vi "extract_para_from_command.vi"(8 "error in (no error)":errorcluster, 11 "Instrument Command In":string=":ACP:OFFS{1|2}:LIST:RCAR {<REAL>}, {<REAL>}, {<REAL>}, {<REAL>}, {<REAL>}, {<REAL>}") -> (0 "error out":errorcluster, 2 "Auto Extracted Contol Specs":T1, 3 "Instrument Command In Out":string)   [LabVIEW 2018]
uses:
  TypeDefinitions/auto_extracted_control_specs.ctl
  TypeDefinitions/auto_extracted_control_spec.ctl
  Gtor/Mth/GenVI/Intf/GenStdVI/Mth/GenOneStdVI/TypeDefinitions/control_data_type.ctl
  Gtor/Mth/GenVI/Intf/GenStdVI/Mth/GenOneStdVI/TypeDefinitions/control_class.ctl
  Gtor/Mth/GenVI/Intf/GenStdVI/Mth/GenOneStdVI/TypeDefinitions/ring_string_and_value.ctl
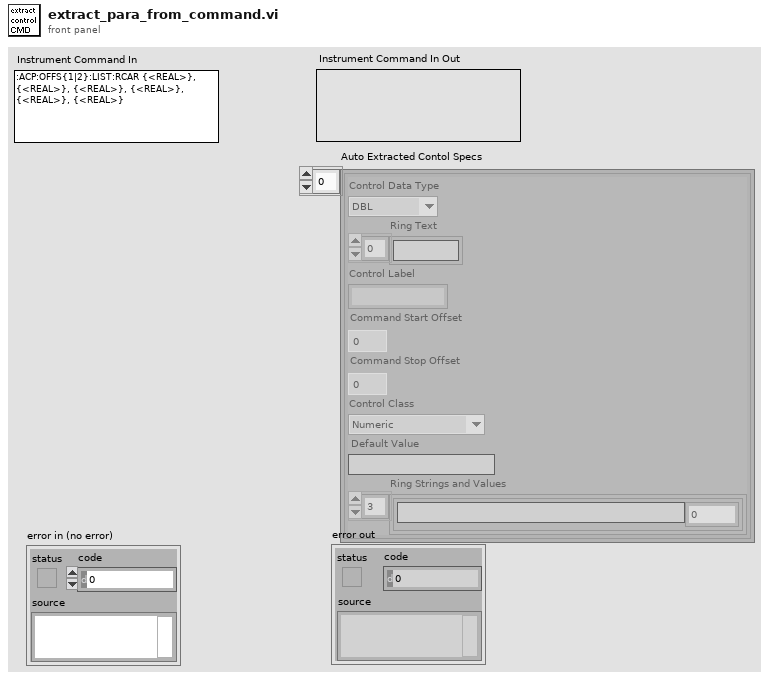
[diagram p1: front panel]
types:
  T1 = typedef "auto_extracted_control_specs.ctl" = T2[]
  T2 = typedef "auto_extracted_control_spec.ctl" = cluster{"Control Data Type":T3, "Ring Text":string[], "Control Label":string, "Command Start Offset":i32, "Command Stop Offset":i32, "Control Class":T4, "Default Value":string, "Ring Strings and Values":T5[]}
  T3 = typedef "control_data_type.ctl" = enum16{"DBL", "I32", "Boolean", "String", "U16", "U32", "EXT", "SGL", "I16", "U8", "I8", "I64", "U64", "Waveform", "Reference", "Variant", "Cluster"}
  T4 = typedef "control_class.ctl" = enum16{"Numeric", "Vertical Slide Switch", "Text Ring", "String", "Array", "VISAName", "WaveformGraph", "Cluster"}
  T5 = typedef "ring_string_and_value.ctl" = cluster{"String":string, "Value":dbl}
  T6 = cluster{"Start Sting":string, "End String":string}
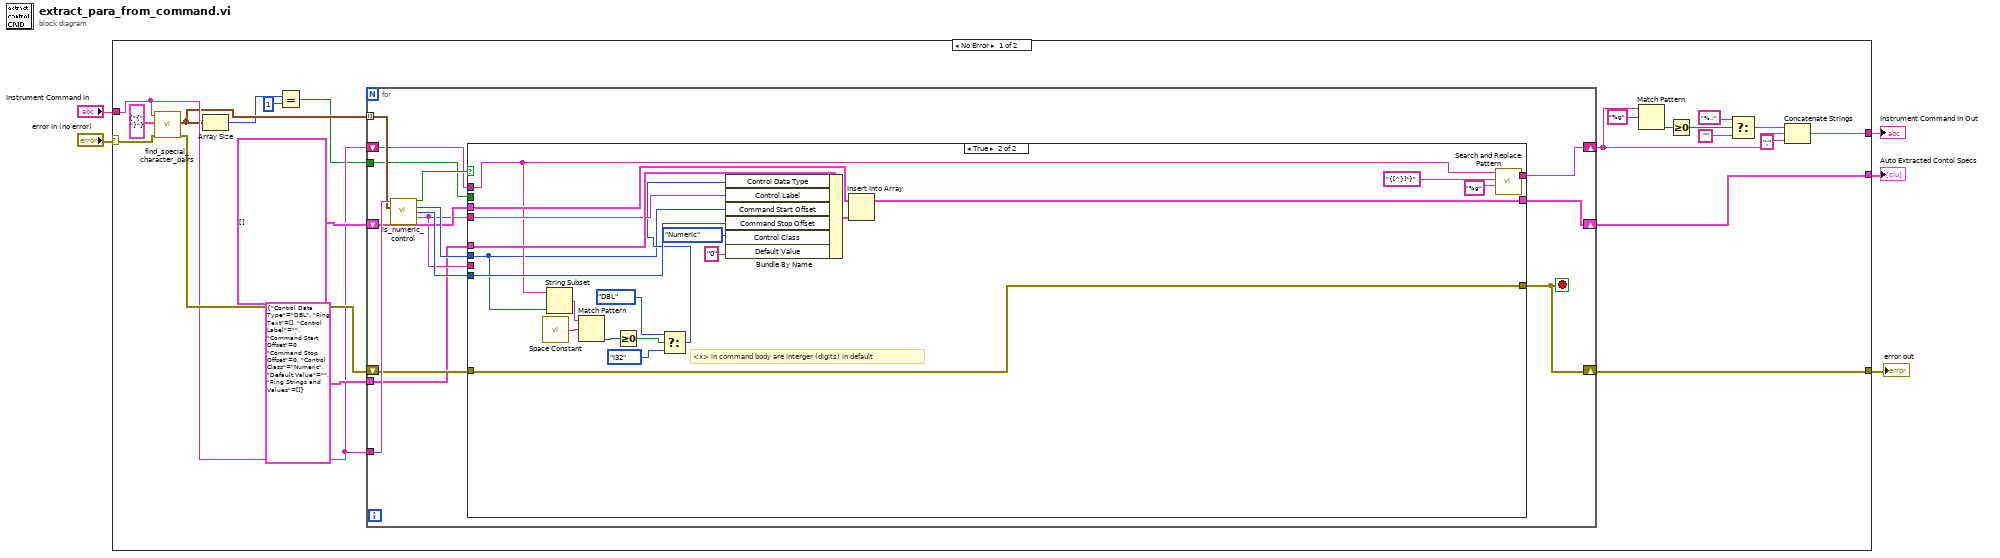
[diagram p0: block diagram]
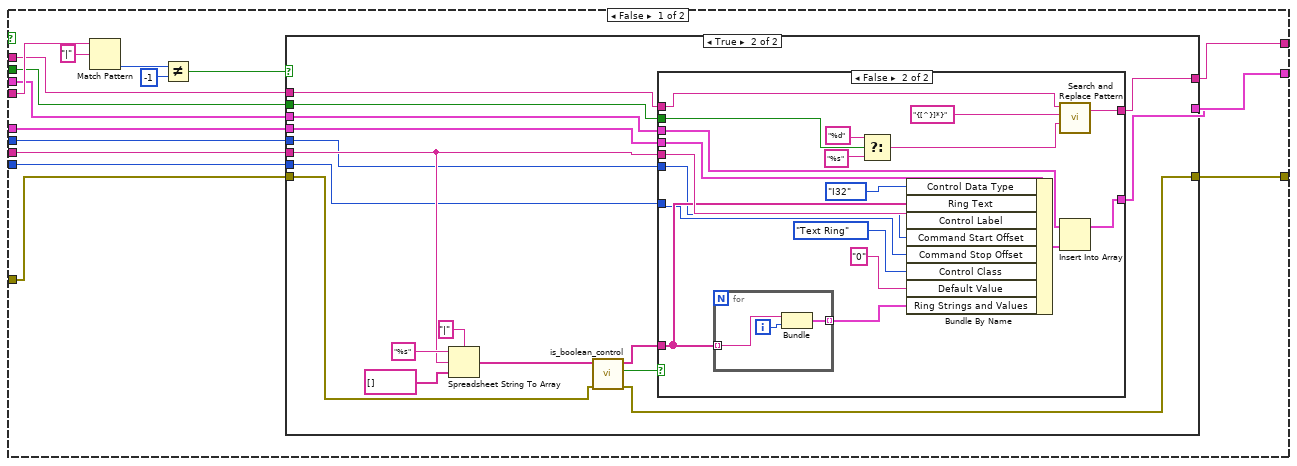
[diagram p2: hidden frame]
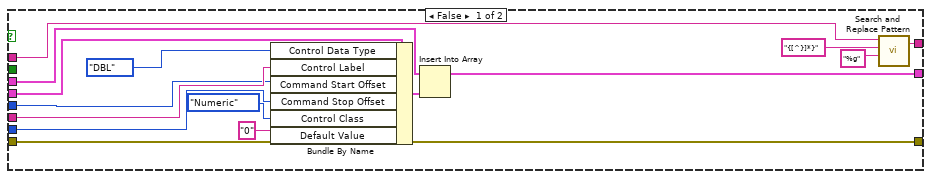
[diagram p3: hidden frame]
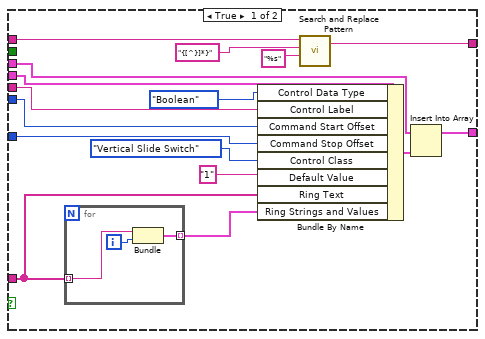
[diagram p4: hidden frame]
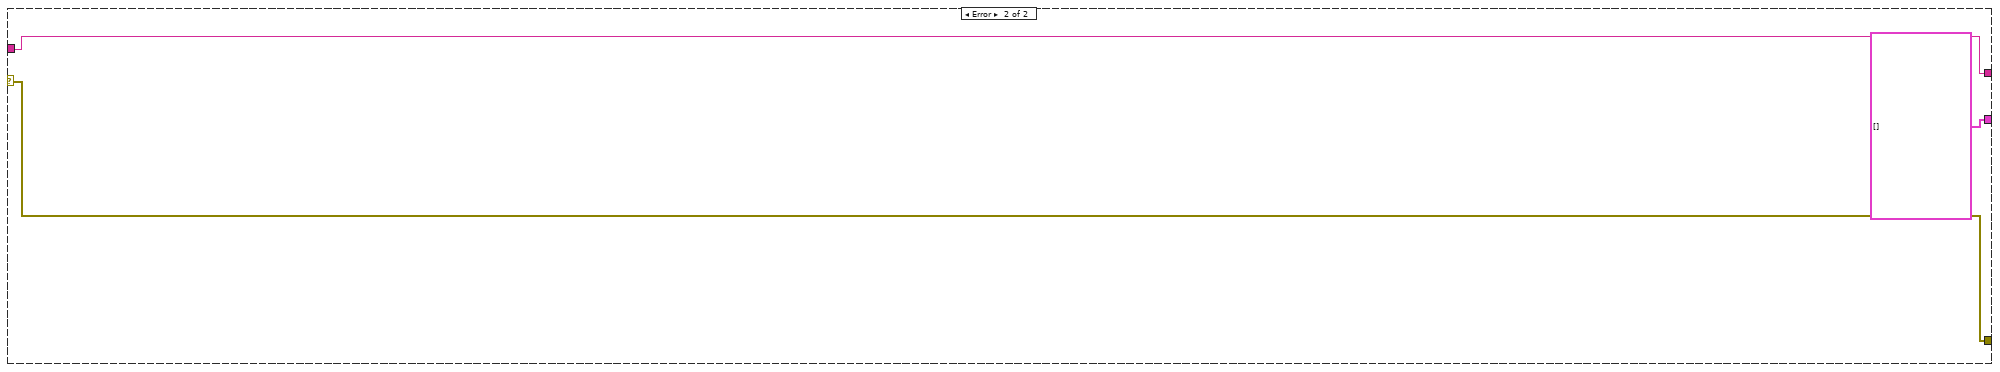
[diagram p5: hidden frame]
diagram:
  n1 = case shown="No Error" "error in (no error)" {
    selector: "error in (no error)" -> [w22 w153]
    tunnel: "Instrument Command In" -> [w19 w151]
    tunnel: [w24 T1 [] ("Auto Extracted Contol Specs")] -> w5
    tunnel: [w23 w153] -> w2
    tunnel: [w11 w151] -> w1
    frame No Error {
      n2 = call "find_special_character_pairs.vi"("error in (no error)"=w22, "String Pair"=T6 {"Start Sting"="{", "End String"="}"}, "Command String"=w19) -> ("error out"=w21:errorcluster, "Pair Offset"=w10:cluster{"Start Offset":i32, "End offset":i32}[])  [unwired: 7 out]
      n3 = Array Size(array=w10) -> (size(s)=w9:i32)
      n4 = Equal?(x=w9, y=1) -> (x = y?=w7:bool)
      n5 = for {
        tunnel: w10 -> [w39] mode=indexing
        tunnel: w19 -> [w40]
        shift-right: [w34] -> w24
        shift-left: T1 [] ("Auto Extracted Contol Specs") -> [w35]
        shift-right: [w27] -> w23
        shift-left: w21 -> [w32]
        tunnel: T2 {"Control Data Type"=enum."DBL", "Ring Text"=[], "Control Label"="", "Command Start Offset"=0, "Command Stop Offset"=0, "Control Class"=enum."Numeric", "Default Value"="", "Ring Strings and Values"=[]} ("Auto Extracted Contol Spec") -> [w31]
        shift-right: [w29] -> w12
        shift-left: w19 -> [w30]
        tunnel: w7 -> [w28]
        stop <- w27 stop-if-true
        n6 = call "is_numeric_control.vi"("Polished Command In"=w40, "Cluster"=w39) -> ("Is Numeric"=w38:bool, "Start Offset"=w37:i32, "End offset"=w36:i32, "Parameter Strings"=w33:string)  [unwired: 1 in, 9 out]
        n7 = case shown="True" w38 {
          tunnel: w33 -> [w55 w146]
          tunnel: w37 -> [w50 w130]
          tunnel: w36 -> [w49 w142]
          tunnel: w35 -> [w48 w150]
          tunnel: [w47 w149] -> w34
          tunnel: w33 -> [w51 _]
          tunnel: w32 -> [w46 w148]
          tunnel: [w45 w148] -> w27
          tunnel: w31 -> [w41 w147]
          tunnel: w30 -> [w44 w133]
          tunnel: [w43 w139] -> w29
          tunnel: w28 -> [w42 _]
          frame False {
            n8 = Match Pattern(string=w55, regular expression="|") -> (offset past match=w54:i32)  [unwired: 4 out]
            n9 = Not Equal?(x=w54, y=-1) -> (x != y?=w52:bool)
            n10 = case shown="True" w52 {
              tunnel: w51 -> [w68 w83]
              tunnel: w50 -> [w59 w82]
              tunnel: w49 -> [w63 w81]
              tunnel: w48 -> [w71 w84]
              tunnel: [w70 w80] -> w47
              tunnel: w46 -> [w69 w78]
              tunnel: [w69 w77] -> w45
              tunnel: w41 -> [w65 w76]
              tunnel: w44 -> [w58 w75]
              tunnel: [w60 w74] -> w43
              tunnel: w42 -> [_ w73]
              frame False {
                n11 = Bundle By Name(cluster=w65, "Control Data Type"=control_data_type."DBL", "Control Label"=w68, "Command Start Offset"=w59, "Command Stop Offset"=w63, "Control Class"=control_class."Numeric", "Default Value"="0") -> (w64:T2)
                n12 = Insert Into Array(array=w71, new element=w64) -> (w70:T1)  [unwired: 1 in]
                n13 = call <vilib>:"Search and Replace Pattern.vi"("string"=w58, "regular expression (\"\")"="{[^}]*}" ("substring (\"\")"), "replace string (\"\")"="%g" ("substring (\"\")")) -> ("result string"=w60:string)  [unwired: 3 out]
              }
              frame True {
                n14 = Spreadsheet String To Array(delimiter (Tab)="|", format string="%s" ("spreadsheet string"), spreadsheet string=w83, array type (2D Dbl)=string[] []) -> (array=w79:string[])
                n15 = call "is_boolean_control.vi"("error in (no error)"=w78, "CMD Ring Value"=w79) -> ("error out"=w77:errorcluster, "Is Boolean"=w85:bool, "CMD Ring Value Out"=w72:string[])  [unwired: 7 out]
                n16 = case shown="False" w85 {
                  tunnel: w84 -> [w104 w126]
                  tunnel: w83 -> [w100 w122]
                  tunnel: w82 -> [w95 w115]
                  tunnel: w81 -> [w96 w116]
                  tunnel: [w103 w125] -> w80
                  tunnel: w72 -> [w90 w120]
                  tunnel: w76 -> [w102 w124]
                  tunnel: w75 -> [w93 w114]
                  tunnel: [w91 w112] -> w74
                  tunnel: w73 -> [_ w111]
                  frame True {
                    n17 = for {
                      tunnel: w90 -> [w107] mode=indexing
                      tunnel: [w105] -> w89 mode=indexing
                      i -> [w106]
                      n18 = Bundle("Ring Value"=w107, w106) -> (w105:cluster{"Ring Value":string, i32})  [unwired: 1 out]
                    }
                    n19 = Bundle By Name(cluster=w102, "Control Data Type"=control_data_type."Boolean", "Control Label"=w100, "Command Start Offset"=w95, "Command Stop Offset"=w96, "Control Class"=control_class."Vertical Slide Switch", "Default Value"="1", "Ring Text"=w90, "Ring Strings and Values"=w89) -> (w98:T2)
                    n20 = call <vilib>:"Search and Replace Pattern.vi"("string"=w93, "regular expression (\"\")"="{[^}]*}" ("substring (\"\")"), "replace string (\"\")"="%s" ("substring (\"\")")) -> ("result string"=w91:string)  [unwired: 3 out]
                    n21 = Insert Into Array(array=w104, new element=w98) -> (w103:T1)  [unwired: 1 in]
                  }
                  frame False {
                    n22 = for {
                      tunnel: w120 -> [w129] mode=indexing
                      tunnel: [w127] -> w119 mode=indexing
                      i -> [w128]
                      n23 = Bundle("Ring Value"=w129, w128) -> (w127:cluster{"Ring Value":string, i32})  [unwired: 1 out]
                    }
                    n24 = Select(t="%d" ("substring (\"\")"), s=w111, f="%s") -> (s? t:f=w109:string)
                    n25 = Bundle By Name(cluster=w124, "Control Data Type"=control_data_type."I32", "Ring Text"=w120, "Control Label"=w122, "Command Start Offset"=w115, "Command Stop Offset"=w116, "Control Class"=control_class."Text Ring", "Default Value"="0", "Ring Strings and Values"=w119) -> (w118:T2)
                    n26 = call <vilib>:"Search and Replace Pattern.vi"("string"=w114, "regular expression (\"\")"="{[^}]*}" ("substring (\"\")"), "replace string (\"\")"=w109) -> ("result string"=w112:string)  [unwired: 3 out]
                    n27 = Insert Into Array(array=w126, new element=w118) -> (w125:T1)  [unwired: 1 in]
                  }
                }
              }
            }
          }
          frame True {
            # "<x> in command body are interger (digits) in default"
            n28 = call <vilib>:"Space Constant.vi"() -> ("String"=w135:string)
            n29 = String Subset(string=w133, length (rest)=w130) -> (substring=w134:string)  [unwired: 1 out]
            n30 = Match Pattern(string=w134, regular expression=w135) -> (offset past match=w136:i32)  [unwired: 4 out]
            n31 = Greater Or Equal To 0?(x=w136) -> (x >= 0?=w137:bool)
            n32 = Select(t=control_data_type."DBL" ("Control Data Type"), s=w137, f=control_data_type."I32" ("Control Data Type")) -> (s? t:f=w131:T3)
            n33 = Bundle By Name(cluster=w147, "Control Data Type"=w131, "Control Label"=w146, "Command Start Offset"=w130, "Command Stop Offset"=w142, "Control Class"=control_class."Numeric", "Default Value"="0") -> (w143:T2)
            n34 = Insert Into Array(array=w150, new element=w143) -> (w149:T1)  [unwired: 1 in]
            n35 = call <vilib>:"Search and Replace Pattern.vi"("string"=w133, "regular expression (\"\")"="{[^}]*}" ("substring (\"\")"), "replace string (\"\")"="%g" ("substring (\"\")")) -> ("result string"=w139:string)  [unwired: 3 out]
          }
        }
      }
      n36 = Match Pattern(string=w12, regular expression="%g") -> (offset past match=w17:i32)  [unwired: 4 out]
      n37 = Greater Or Equal To 0?(x=w17) -> (x >= 0?=w16:bool)
      n38 = Select(t="%.;", s=w16, f="") -> (s? t:f=w13:string)
      n39 = Concatenate Strings(w13, w12, ";" ("string")) -> (w11:string)
    }
    frame Error {
    }
  }
  "Auto Extracted Contol Specs" <- w5
  "error out" <- w2
  "Instrument Command In Out" <- w1
